vi "Add_spot_dialog_old.vi"(7 "Modify":bool, 8 "TransformedPt":bool, 9 "ArrayOfSpotNames":string[](array[string]), 10 "Current Session Information":T1={"CollectionOfPoints"=[{"MetaDataFile"=path "", "X"=0.0, "Y"=0.0, "Z"=0.0, "Group"=0, "Rotation"=0.0, "Fiducial"=FALSE, "Magnification"=0.0, "Working_Distance"=0.0, "Notes"="", "Location Name/ID"="", "OtherRelatedDataFiles"=[], "Available"=FALSE}, {"MetaDataFile"=path "", "X"=0.0, "Y"=0.0, "Z"=0.0, "Group"=0, "Rotation"=0.0, "Fiducial"=FALSE, "Magnification"=0.0, "Working_Distance"=0.0, "Notes"="", "Location Name/ID"="", "OtherRelatedDataFiles"=[], "Available"=FALSE}, {"MetaDataFile"=path "", "X"=0.0, "Y"=0.0, "Z"=0.0, "Group"=0, "Rotation"=0.0, "Fiducial"=FALSE, "Magnification"=0.0, "Working_Distance"=0.0, "Notes"="", "Location Name/ID"="", "OtherRelatedDataFiles"=[], "Available"=FALSE}, {"MetaDataFile"=path "", "X"=0.0, "Y"=0.0, "Z"=0.0, "Group"=0, "Rotation"=0.0, "Fiducial"=FALSE, "Magnification"=0.0, "Working_Distance"=0.0, "Notes"="", "Location Name/ID"="", "OtherRelatedDataFiles"=[], "Available"=FALSE}, {"MetaDataFile"=path "", "X"=0.0, "Y"=0.0, "Z"=0.0, "Group"=0, "Rotation"=0.0, "Fiducial"=FALSE, "Magnification"=0.0, "Working_Distance"=0.0, "Notes"="", "Location Name/ID"="", "OtherRelatedDataFiles"=[], "Available"=FALSE}, {"MetaDataFile"=path "", "X"=0.0, "Y"=0.0, "Z"=0.0, "Group"=0, "Rotation"=0.0, "Fiducial"=FALSE, "Magnification"=0.0, "Working_Distance"=0.0, "Notes"="", "Location Name/ID"="", "OtherRelatedDataFiles"=[], "Available"=FALSE}, {"MetaDataFile"=path "", "X"=0.0, "Y"=0.0, "Z"=0.0, "Group"=0, "Rotation"=0.0, "Fiducial"=FALSE, "Magnification"=0.0, "Working_Distance"=0.0, "Notes"="", "Location Name/ID"="", "OtherRelatedDataFiles"=[], "Available"=FALSE}], "Instrument"=enum."MXRD MFC", "CollectionFile"=path "/INL Macintosh/Users/timothymcjunkin/Desktop/Diffusion couple/MXRD 9-13-10/xrd_session_for_corrected.xml", "Session Name/ID"="xrd_test", "SessionNotes"="Sample moved to XRD"}, 11 "Input of Spot information":T2) -> (0 "Output of Spot information":T2, 1 "Current Session Information Out":T1={"CollectionOfPoints"=[{"MetaDataFile"=path "", "X"=0.0, "Y"=0.0, "Z"=0.0, "Group"=0, "Rotation"=0.0, "Fiducial"=FALSE, "Magnification"=0.0, "Working_Distance"=0.0, "Notes"="", "Location Name/ID"="", "OtherRelatedDataFiles"=[], "Available"=FALSE}, {"MetaDataFile"=path "", "X"=0.0, "Y"=0.0, "Z"=0.0, "Group"=0, "Rotation"=0.0, "Fiducial"=FALSE, "Magnification"=0.0, "Working_Distance"=0.0, "Notes"="", "Location Name/ID"="", "OtherRelatedDataFiles"=[], "Available"=FALSE}, {"MetaDataFile"=path "", "X"=0.0, "Y"=0.0, "Z"=0.0, "Group"=0, "Rotation"=0.0, "Fiducial"=FALSE, "Magnification"=0.0, "Working_Distance"=0.0, "Notes"="", "Location Name/ID"="", "OtherRelatedDataFiles"=[], "Available"=FALSE}, {"MetaDataFile"=path "", "X"=0.0, "Y"=0.0, "Z"=0.0, "Group"=0, "Rotation"=0.0, "Fiducial"=FALSE, "Magnification"=0.0, "Working_Distance"=0.0, "Notes"="", "Location Name/ID"="", "OtherRelatedDataFiles"=[], "Available"=FALSE}, {"MetaDataFile"=path "", "X"=0.0, "Y"=0.0, "Z"=0.0, "Group"=0, "Rotation"=0.0, "Fiducial"=FALSE, "Magnification"=0.0, "Working_Distance"=0.0, "Notes"="", "Location Name/ID"="", "OtherRelatedDataFiles"=[], "Available"=FALSE}, {"MetaDataFile"=path "", "X"=0.0, "Y"=0.0, "Z"=0.0, "Group"=0, "Rotation"=0.0, "Fiducial"=FALSE, "Magnification"=0.0, "Working_Distance"=0.0, "Notes"="", "Location Name/ID"="", "OtherRelatedDataFiles"=[], "Available"=FALSE}, {"MetaDataFile"=path "", "X"=0.0, "Y"=0.0, "Z"=0.0, "Group"=0, "Rotation"=0.0, "Fiducial"=FALSE, "Magnification"=0.0, "Working_Distance"=0.0, "Notes"="", "Location Name/ID"="", "OtherRelatedDataFiles"=[], "Available"=FALSE}], "Instrument"=enum."MXRD MFC", "CollectionFile"=path "/INL Macintosh/Users/timothymcjunkin/Desktop/Diffusion couple/MXRD 9-13-10/xrd_session_for_corrected.xml", "Session Name/ID"="xrd_test", "SessionNotes"="Sample moved to XRD"}, 3 "Cancel":bool)   [LabVIEW 2011]
doc: "Pressing any of the add modify spots buttons launches a multi-purpose dialog box which is reconfigured to parts of the dialog box the user interacts with in each mode. This effectively reuses a lot of code that would have needed to be duplicated for the different cases. In the process makes this one dialog box more complicated. This dialog also gets called after a spot from a previous session dialog box is completed. Two types of adds are possible without a calculation, one for a fiducial and one for a spot of interest that is not a fiducial. The modify version of this dialog box is simply supplied with the exiting information from a spot and allows the user to change the spot information. It may be called from the modify or the edit button on the sample information tab or the current session tab. The only difference is where the information comes from and goes to."
uses:
  cm2nm_coordinate_information_v2.ctl
  cm2nm_sample_set.ctl
  Instrument_type_enum_v2.ctl
  cm2nm_fiducial_selector.ctl
panel:
  in  "Allow_nonstandard_fids":bool
  out "error out 2":errorcluster
  in  "Cancel 2":bool
  out "Original_group":i32
  out "Instructions":string
  in  "Group Coding":i32
  out "MetaDataAvailable":bool caption="Is a Fiducial"
  out "error out":errorcluster
  in  "Notes:":string
  in  "Tab Control":T4(tab)
  in  "Fiducial Selector":T5
  in  "Tilt":dbl
  in  "Stage Rotation":dbl
  in  "Get Coordinates from Meta File":bool
  in  "Move to next screen":bool
  in  "Spot Name":string
  in  "Z-Position":dbl
  in  "Y-Position":dbl
  in  "X-Position":dbl
  in  "MetaDataFile":path
  in  "Cancel2":bool caption="Cancel"
  in  "Fiducial?":bool
  in  "Add A Spot Related Data File":bool caption="Add Another File\nRelated to this Spot"
  in  "Goto Previous Screen":bool caption="Press to Move to \nPrevious Screen"
  in  "Press to goto final Screen":bool caption="Press to Move to Next\nInformation Screen"
  out "OtherRelatedDataFiles":T6(array[cluster])
  in  "Cancel3":bool
  in  "Go Back to Correct":bool
  in  "AddToDataBase":bool
  # "Enter or confirm the\nspot  name and positions\n\nIf Metafile is available \nselect it in the MetaDatafile\nField and click Use MetaFile\nto extract MetaData\nFrom the file."
  # "This form allows you\nto add any number of\nfiles related to this\nspot on the sample.\nFor example spectra\nfiles or images other\nthan the file \ncontaining meta data."
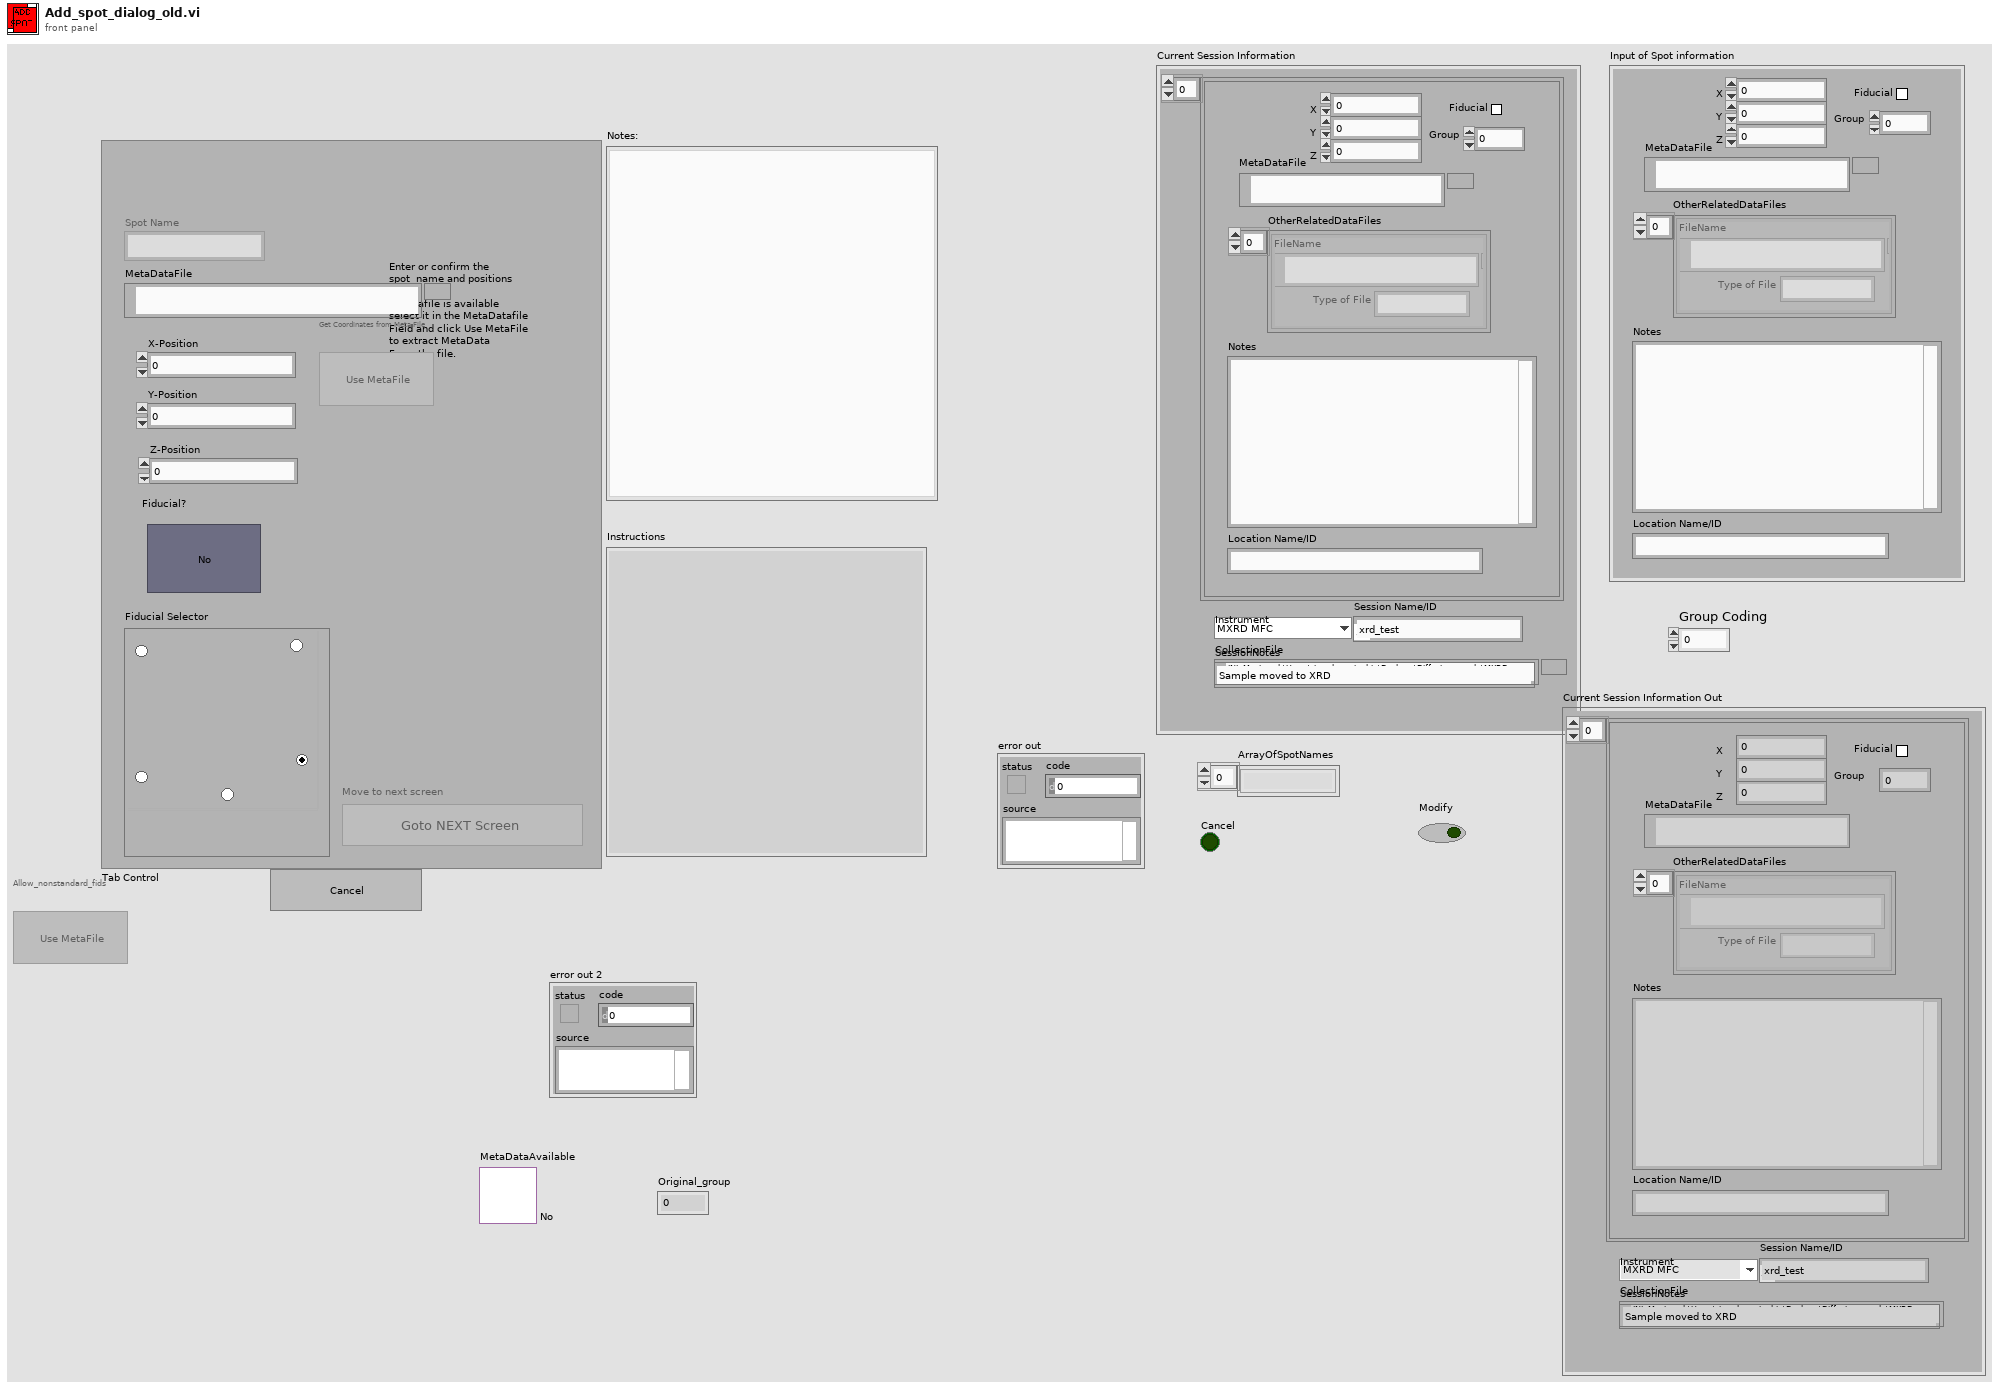
[diagram p1: front panel]
types:
  T1 = typedef "cm2nm_sample_set.ctl" = cluster{"CollectionOfPoints":T2[], "Instrument":T3, "CollectionFile":path, "Session Name/ID":string, "SessionNotes":string}
  T2 = typedef "cm2nm_coordinate_information_v2.ctl" = cluster{"MetaDataFile":path, "X":dbl, "Y":dbl, "Z":dbl, "Group":i32, "Rotation":dbl[unit], "Fiducial":bool, "Magnification":dbl, "Working_Distance":dbl, "Notes":string, "Location Name/ID":string, "OtherRelatedDataFiles":cluster{"Type of File":string, "FileName":path}[], "Available":bool}
  T3 = typedef "Instrument_type_enum_v2.ctl" = enum16{"Unknown", "Philips FEI SEM IRC", "JEOL 7000F EML_MFC", "MXRD MFC", "JEOL_EPMA"}
  T4 = enum32{"Name and Postions", "ExtraDataFiles", "SpotSummary"}
  T5 = typedef "cm2nm_fiducial_selector.ctl" = enum32{"Fiducial 1", "Fiducial 2", "Fiducial 3", "Fiducial 4", "Fiducial 5", "Other/NonStandard"}
  T6 = cluster{"Type of File":string, "FileName":path}[]
  T7 = enum8{"Enabled", "Disabled", "Disabled and Grayed Out"}
  T8 = enum32{"Name and Postions", "ExtraDataFiles", "SpotSummary", "Inputs"}
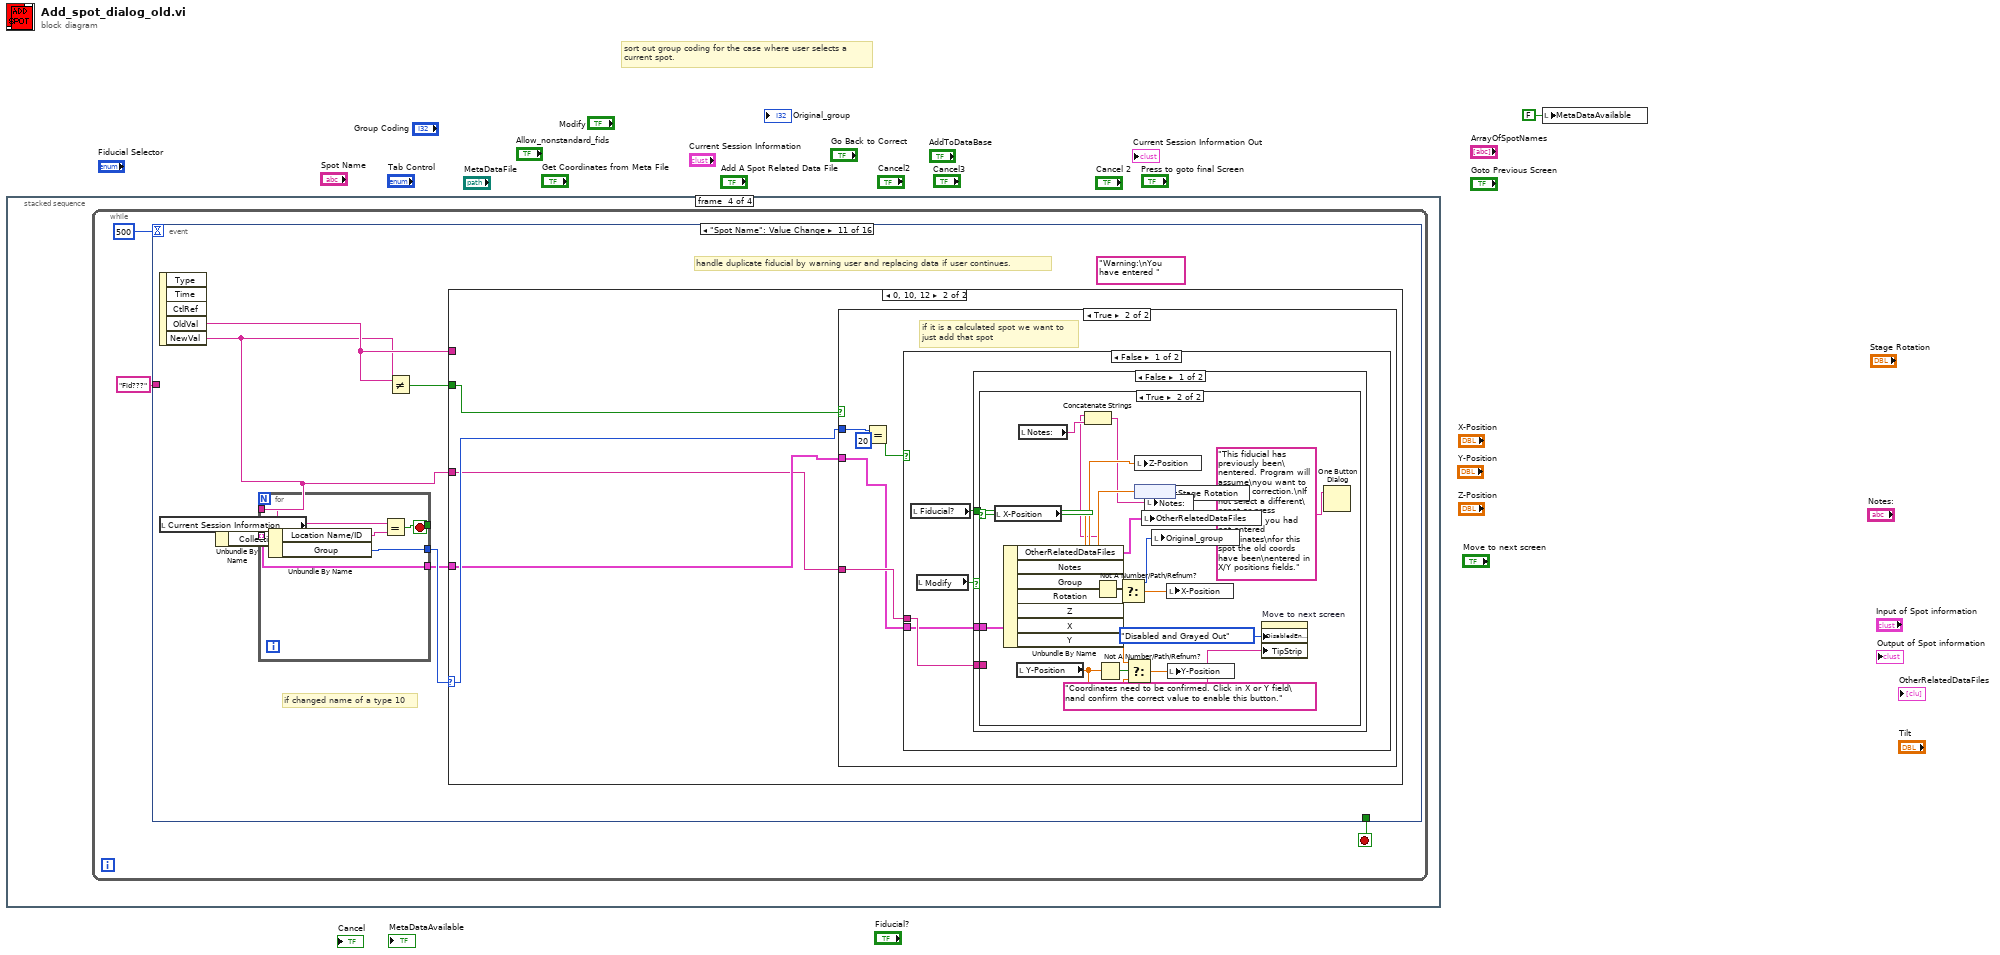
[diagram p0: block diagram]
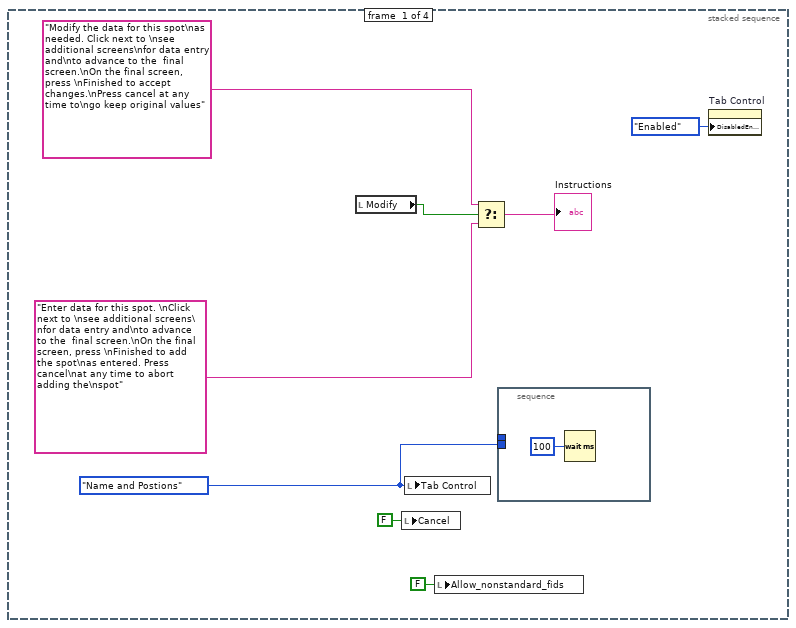
[diagram p2: hidden frame]
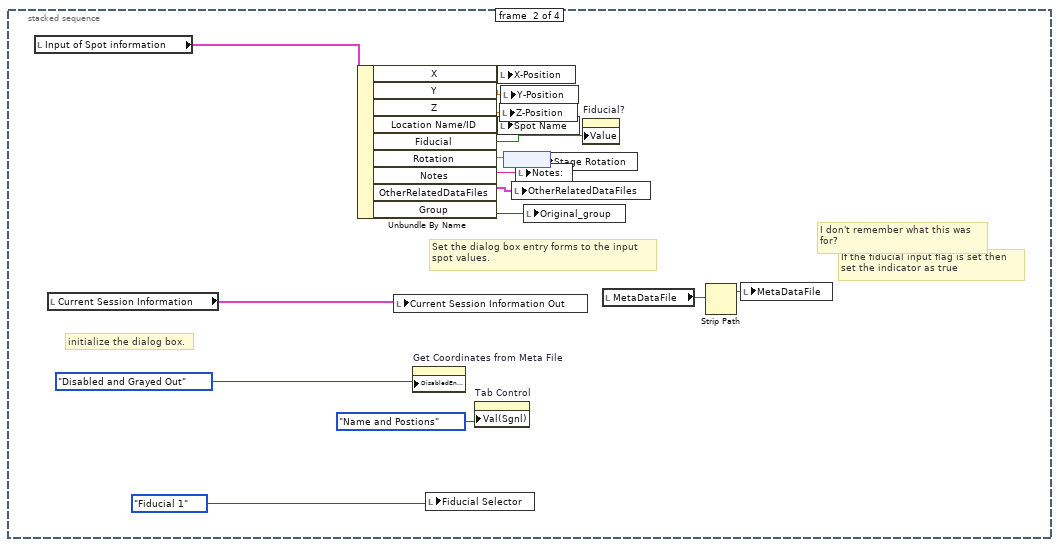
[diagram p3: hidden frame]
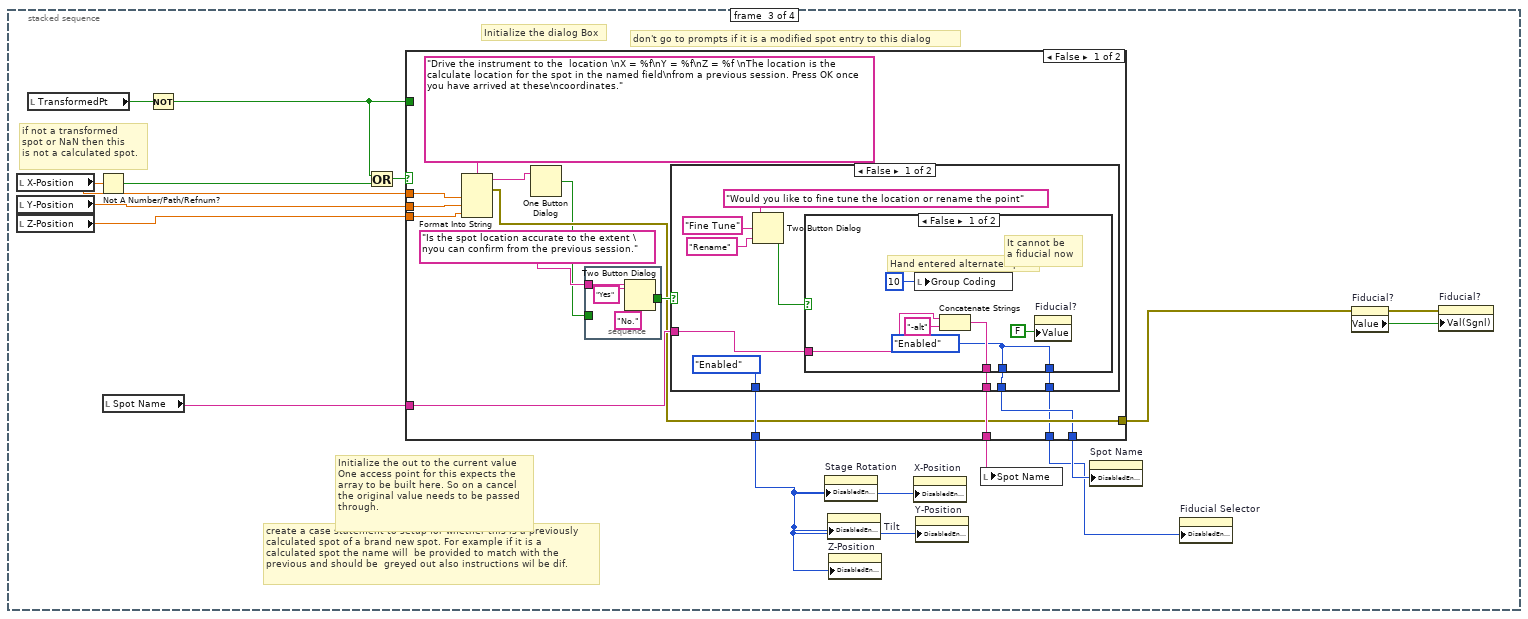
[diagram p4: hidden frame]
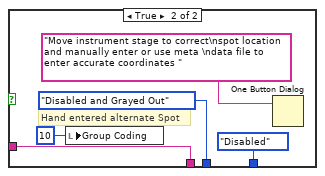
[diagram p5: hidden frame]
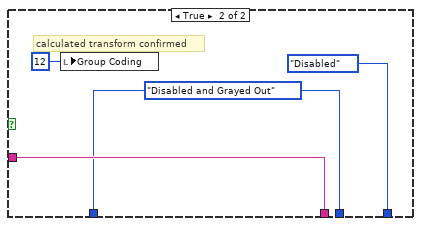
[diagram p6: hidden frame]
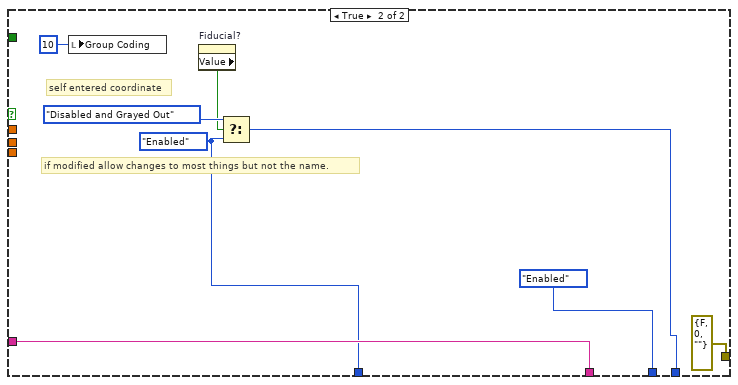
[diagram p7: hidden frame]
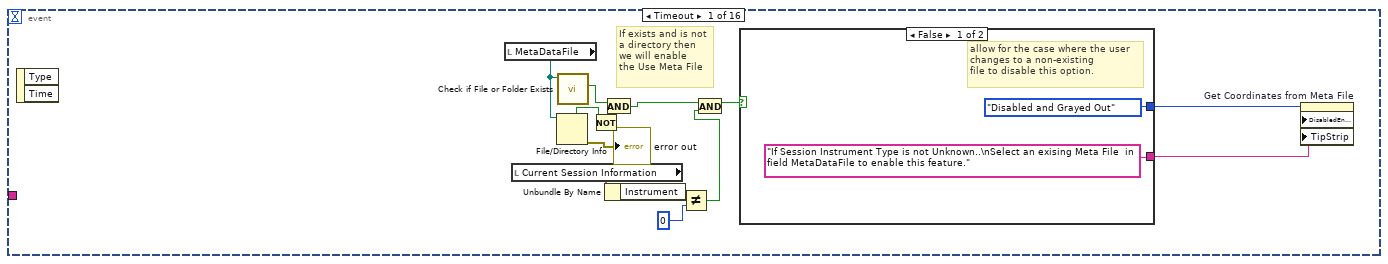
[diagram p8: hidden frame]
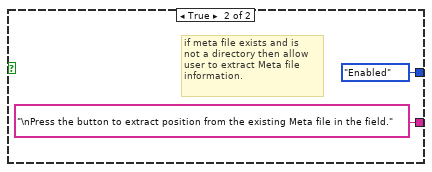
[diagram p9: hidden frame]
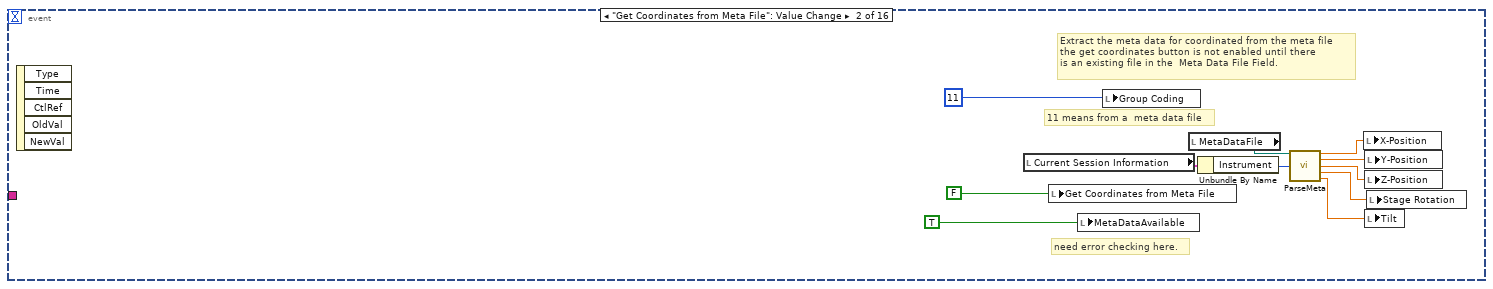
[diagram p10: hidden frame]
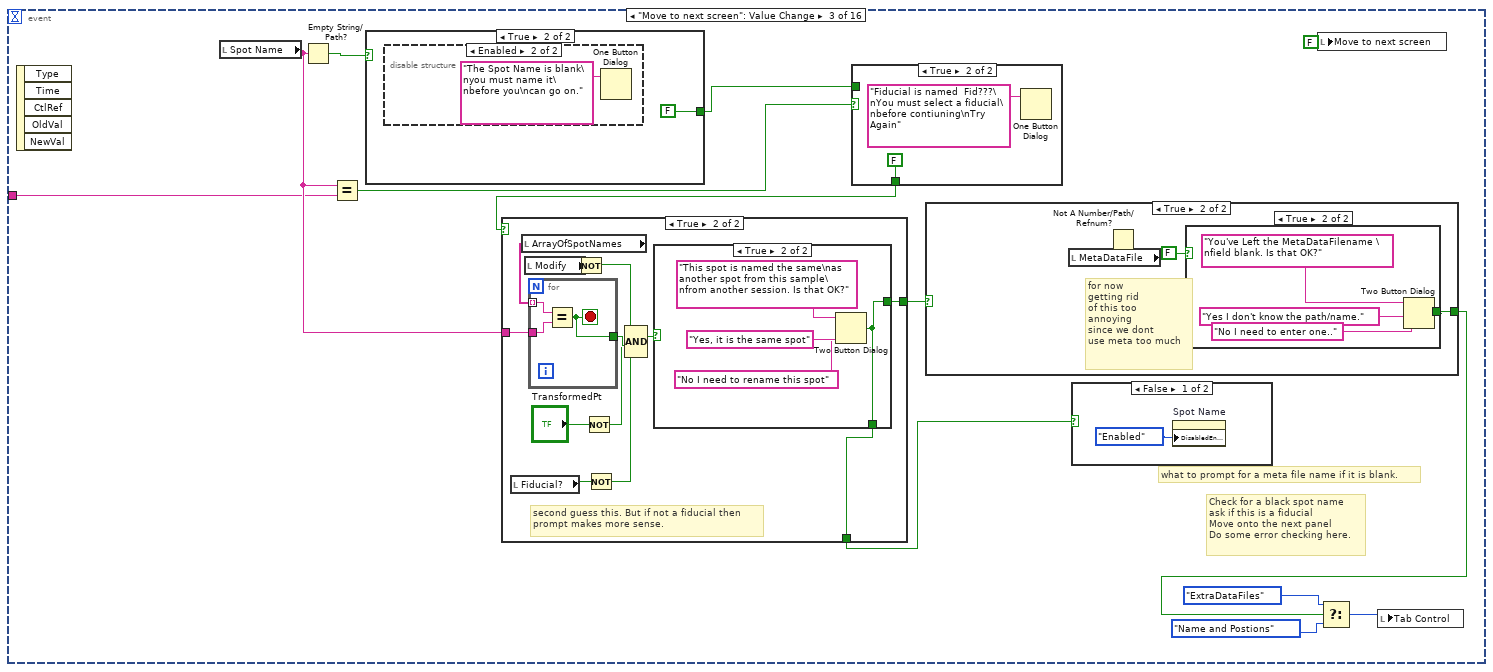
[diagram p11: hidden frame]
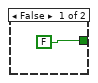
[diagram p14: hidden frame]
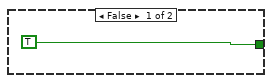
[diagram p15: hidden frame]
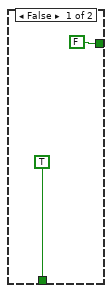
[diagram p16: hidden frame]
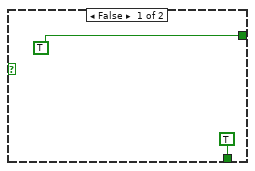
[diagram p17: hidden frame]
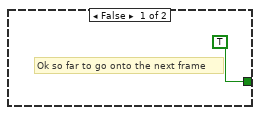
[diagram p18: hidden frame]
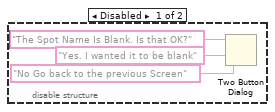
[diagram p19: hidden frame]
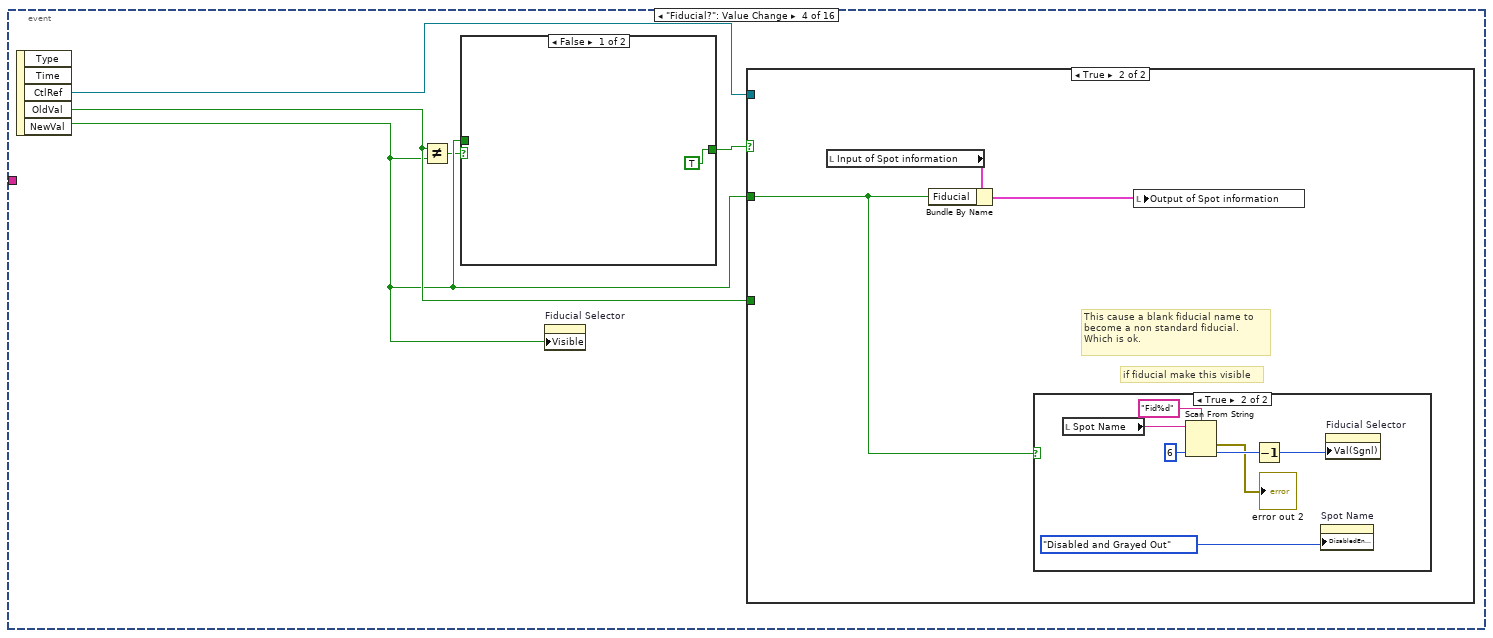
[diagram p20: hidden frame]
diagram:
  # "sort out group coding for the case where user selects a\ncurrent spot."
  n1 = stacked-sequence {
    frame #0 {
      w5 = T8."Name and Postions" ("Tab Control")
      n2 = local read "Modify"() -> (w6:bool)
      n3 = local write "Cancel"(FALSE ("Cancel")) -> ()
      n4 = local write "Tab Control"(w5) -> ()
      n5 = local write "Allow_nonstandard_fids"(FALSE ("Allow_nonstandard_fids")) -> ()
      n6 = Select(t="Modify the data for this spot\nas needed. Click next to \nsee additional screens\nfor data entry and\nto advance to the  final screen.\nOn the final screen, press \nFinished to accept changes.\nPress cancel at any time to\ngo keep original values" ("Instructions"), s=w6, f="Enter data for this spot. \nClick next to \nsee additional screens\nfor data entry and\nto advance to the  final screen.\nOn the final screen, press \nFinished to add the spot\nas entered. Press cancel\nat any time to abort adding the\nspot" ("Instructions")) -> (s? t:f=→"Instructions":string)
      n7 = stacked-sequence {
        tunnel: [w10] -> _
        tunnel: w5 -> [w10]
        frame #0 {
          n8 = Wait (ms)(milliseconds to wait=u32 100) -> ()  [unwired: 1 out]
        }
      }
      n9 = property on="Tab Control" class="TabCtl (strict)"("DisabledEnum"=T7."Enabled" ("Disabled")) -> ()  [unwired: 2 in, 2 out]
    }
    frame #1 {
      # "initialize the dialog box."
      # "I don't remember what this was\nfor?"
      # "If the fiducial input flag is set then \nset the indicator as true"
      # "Set the dialog box entry forms to the input\nspot values."
      n10 = local read "Input of Spot information"() -> (w28:T2)
      n11 = local read "Current Session Information"() -> (w19:T1)
      n12 = Unbundle By Name(w28) -> ("X"=w20:dbl, "Y"=w27:dbl, "Z"=w25:dbl, "Location Name/ID"=w26:string, "Fiducial"=w14:bool, "Rotation"=w24:dbl[unit], "Notes"=w22:string, "OtherRelatedDataFiles"=w21:T6, "Group"=w12:i32)
      n13 = local write "Current Session Information Out"(w19) -> ()
      n14 = property on="Get Coordinates from Meta File" class="Bool (strict)"("DisabledEnum"=T7."Disabled and Grayed Out" ("Disabled")) -> ()  [unwired: 2 in, 2 out]
      n15 = local write "Fiducial Selector"(cm2nm_fiducial_selector."Fiducial 1" ("Fiducial Selector")) -> ()
      n16 = property on="Tab Control" class="TabCtl (strict)"("Val(Sgnl)"=T8."Name and Postions" ("Tab Control")) -> ()  [unwired: 2 in, 2 out]
      n17 = local write "X-Position"(w20) -> ()
      n18 = local write "Spot Name"(w26) -> ()
      n19 = local write "Z-Position"(w25) -> ()
      n20 = local write "Y-Position"(w27) -> ()
      n21 = node(w24) -> (w23:dbl)
      n22 = local write "OtherRelatedDataFiles"(w21) -> ()
      n23 = local write "Notes:"(w22) -> ()
      n24 = local write "Original_group"(w12) -> ()
      n25 = local write "Stage Rotation"(w23) -> ()
      n26 = property on="Fiducial?" class="Bool (strict)"("Value"=w14) -> ()  [unwired: 2 in, 2 out]
      n27 = local read "MetaDataFile"() -> (w16:path)
      n28 = Strip Path(path=w16) -> (stripped path=w15:path)  [unwired: 1 out]
      n29 = local write "MetaDataFile"(w15) -> ()
    }
    frame #2 {
      # "if not a transformed\nspot or NaN then this\nis not a calculated spot."
      # "don't go to prompts if it is a modified spot entry to this dialog"
      # "Initialize the out to the current value\nOne access point for this expects the\narray to be built here. So on a cancel\nthe original value needs to be passed\nthrough."
      # "Initialize the dialog Box"
      # "create a case statement to setup for whether this is a previously\ncalculated spot of a brand new spot. For example if it is a\ncalculated spot the name will  be provided to match with the \nprevious and should be  greyed out also instructions wil be dif."
      n30 = local read "X-Position"() -> (w38:dbl)
      n31 = local read "Y-Position"() -> (w40:dbl)
      n32 = local read "Z-Position"() -> (w39:dbl)
      n33 = local read "TransformedPt"() -> (w31:bool)
      n34 = Not A Number/Path/Refnum?(number/path/refnum=w38) -> (NaN/Path/Refnum?=w36:bool)
      n35 = local read "Spot Name"() -> (w37:string)
      n36 = Not(x=w31) -> (.not. x?=w35:bool)
      n37 = Or(x=w35, y=w36) -> (x .or. y?=w41:bool)
      n38 = case shown="False" w41 {
        tunnel: [w50 w89] -> w43
        tunnel: w38 -> [w56 _]
        tunnel: w40 -> [w55 _]
        tunnel: [w45 w90] -> w30
        tunnel: w37 -> [w49 w93]
        tunnel: [w48 w93] -> w42
        tunnel: w39 -> [w52 _]
        tunnel: w35 -> [_ _]
        tunnel: [w47 errorcluster {"status"=FALSE, "code"=0, "source"=""} ("error IO")] -> w33
        tunnel: [w44 T7."Enabled" ("Disabled")] -> w29
        frame False {
          n39 = Format Into String(format string="Drive the instrument to the  location \nX = %f\nY = %f\nZ = %f \nThe location is the calculate location for the spot in the named field\nfrom a previous session. Press OK once you have arrived at these\ncoordinates.", w56, w55, w52) -> (resulting string=w54:string, error out=w47:errorcluster)  [unwired: 2 in]
          n40 = One Button Dialog ("Drive to the Calculated Coordinates")(message=w54) -> (true=w46:bool)  [unwired: 1 in]
          n41 = stacked-sequence {
            tunnel: "Is the spot location accurate to the extent \nyou can confirm from the previous session." -> [w61]
            tunnel: [w58] -> w51
            tunnel: w46 -> [_]
            frame #0 {
              n42 = Two Button Dialog(message=w61, 1:"No." ("F button name (\"Cancel\")"), 2:"Yes" ("T button name (\"OK\")")) -> (T button?=w58:bool)
            }
          }
          n43 = case shown="False" w51 {
            tunnel: [T7."Enabled" ("Disabled") w84] -> w50
            tunnel: w49 -> [w65 w85]
            tunnel: [w64 w85] -> w48
            tunnel: [w63 w84] -> w45
            tunnel: [w62 T7."Disabled" ("Disabled")] -> w44
            frame False {
              n44 = Two Button Dialog(message="Would you like to fine tune the location or rename the point", 1:"Rename" ("F button name (\"Cancel\")"), 2:"Fine Tune" ("T button name (\"OK\")")) -> (T button?=w66:bool)
              n45 = case shown="False" w66 {
                tunnel: w65 -> [w75 w81]
                tunnel: [w74 w81] -> w64
                tunnel: [w71 T7."Disabled and Grayed Out" ("Disabled")] -> w63
                tunnel: [w71 T7."Disabled" ("Disabled")] -> w62
                frame False {
                  w71 = T7."Enabled" ("Disabled")
                  # "It cannot be\na fiducial now"
                  # "Hand entered alternate Spot"
                  n46 = local write "Group Coding"(10 ("Group Coding")) -> ()
                  n47 = Concatenate Strings(w75, "-alt" ("string")) -> (w74:string)
                  n48 = property on="Fiducial?" class="Bool (strict)"("Value"=FALSE ("Fiducial?")) -> ()  [unwired: 2 in, 2 out]
                }
                frame True {
                  # "Hand entered alternate Spot"
                  n49 = local write "Group Coding"(10 ("Group Coding")) -> ()
                  n50 = One Button Dialog ("Drive to the Calculated Coordinates")(message="Move instrument stage to correct\nspot location and manually enter or use meta \ndata file to enter accurate coordinates ") -> ()  [unwired: 1 in, 1 out]
                }
              }
            }
            frame True {
              w84 = T7."Disabled and Grayed Out" ("Disabled")
              # "calculated transform confirmed"
              n51 = local write "Group Coding"(12 ("Group Coding")) -> ()
            }
          }
        }
        frame True {
          w89 = T7."Enabled" ("Disabled")
          # "if modified allow changes to most things but not the name."
          # "self entered coordinate"
          n52 = local write "Group Coding"(10 ("Group Coding")) -> ()
          n53 = property on="Fiducial?" class="Bool (strict)"() -> ("Value"=w87:bool)  [unwired: 2 in, 2 out]
          n54 = Select(t=T7."Disabled and Grayed Out" ("Disabled"), s=w87, f=w89) -> (s? t:f=w90:T7)
        }
      }
      n55 = property on="Stage Rotation" class="DigNum (strict)"("DisabledEnum"=w43) -> ()  [unwired: 2 in, 2 out]
      n56 = property on="Tilt" class="DigNum (strict)"("DisabledEnum"=w43) -> ()  [unwired: 2 in, 2 out]
      n57 = property on="Z-Position" class="DigNum (strict)"("DisabledEnum"=w43) -> ()  [unwired: 2 in, 2 out]
      n58 = property on="X-Position" class="DigNum (strict)"("DisabledEnum"=w43) -> ()  [unwired: 2 in, 2 out]
      n59 = property on="Y-Position" class="DigNum (strict)"("DisabledEnum"=w43) -> ()  [unwired: 2 in, 2 out]
      n60 = local write "Spot Name"(w42) -> ()
      n61 = property on="Spot Name" class="Str"("DisabledEnum"=w30) -> ()  [unwired: 2 in, 2 out]
      n62 = property on="Fiducial Selector" class="RadioBtnsControl (strict)"("DisabledEnum"=w29) -> ()  [unwired: 2 in, 2 out]
      n63 = property on="Fiducial?" class="Bool (strict)"(error in=w33) -> (error out=w34:errorcluster, "Value"=w32:bool)  [unwired: 1 in, 1 out]
      n64 = property on="Fiducial?" class="Bool (strict)"(error in=w34, "Val(Sgnl)"=w32) -> ()  [unwired: 1 in, 2 out]
    }
    frame #3 {
      n65 = while {
        stop <- w95 stop-if-true
        n66 = event shown="[10] \"Spot Name\": Value Change" {
          selector: _ -> [_ _ _ _ _ _ _ _ _ _ _ _ _ _ _ _]
          dyn-events: _ -> [_ _ _ _ _ _ _ _ _ _ _ _ _ _ _ _]
          timeout: 500 -> [_ _ _ _ _ _ _ _ _ _ _ _ _ _ _ _]
          tunnel: [_ _ _ _ _ TRUE ("T button?") w250 _ _ _ _ w362 _ _ _ _] -> w95
          tunnel: "Fid???" ("Value (Signaling)") -> [_ _ w128 _ w206 _ _ _ _ _ _ _ _ _ _ _]
          event Timeout {
            # "If exists and is not\na directory then\nwe will enable \nthe Use Meta File"
            n67 = event-data() -> ()  [unwired: 1 in, 2 out]
            n68 = local read "MetaDataFile"() -> (w102:path)
            n69 = local read "Current Session Information"() -> (w101:T1)
            n70 = File/Directory Info(path=w102) -> (directory=w109:bool, error out=→"error out":errorcluster)  [unwired: 1 in, 5 out]
            n71 = call <vilib>:"Check if File or Folder Exists.vi"("path"=w102) -> ("file or folder exists?"=w107:bool)  [unwired: 8 in, 2 out]
            n72 = Not(x=w109) -> (.not. x?=w108:bool)
            n73 = And(x=w107, y=w108) -> (x .and. y?=w103:bool)
            n74 = Unbundle By Name(w101) -> ("Instrument"=w100:T3)
            n75 = Not Equal?(x=w100, y=u16 0) -> (x != y?=w97:bool)
            n76 = And(x=w103, y=w97) -> (x .and. y?=w98:bool)
            n77 = case shown="False" w98 {
              tunnel: [T7."Disabled and Grayed Out" ("Disabled") T7."Enabled" ("Disabled")] -> w105
              tunnel: ["If Session Instrument Type is not Unknown..\nSelect an exising Meta File  in field MetaDataFile to enable this feature." ("Tip Strip") "\nPress the button to extract position from the existing Meta file in the field." ("Tip Strip")] -> w104
              frame False {
                # "allow for the case where the user\nchanges to a non-existing\nfile to disable this option."
              }
              frame True {
                # "if meta file exists and is\nnot a directory then allow \nuser to extract Meta file \ninformation."
              }
            }
            n78 = property on="Get Coordinates from Meta File" class="Bool (strict)"("DisabledEnum"=w105, "TipStrip"=w104) -> ()  [unwired: 2 in, 2 out]
          }
          event "Get Coordinates from Meta File": Value Change {
            # "11 means from a  meta data file"
            # "need error checking here."
            # "Extract the meta data for coordinated from the meta file\nthe get coordinates button is not enabled until there\nis an existing file in the  Meta Data File Field."
            n79 = event-data() -> ()  [unwired: 1 in, 5 out]
            n80 = local read "Current Session Information"() -> (w115:T1)
            n81 = local write "Get Coordinates from Meta File"(FALSE ("Get Coords")) -> ()
            n82 = local write "MetaDataAvailable"(TRUE ("MetaDataAvailable")) -> ()
            n83 = local write "Group Coding"(11 ("Group Coding")) -> ()
            n84 = local read "MetaDataFile"() -> (w123:path)
            n85 = Unbundle By Name(w115) -> ("Instrument"=w122:T3)
            n86 = call "ParseMeta.vi"("Path"=w123, "Instrument"=w122) -> ("X-stage (um)"=w121:dbl, "Y-stage (um)"=w120:dbl, "Z-stage (um)"=w119:dbl, "R-stage (deg)"=w118:dbl, "StageTilt"=w117:dbl)  [unwired: 1 in, 8 out]
            n87 = local write "X-Position"(w121) -> ()
            n88 = local write "Y-Position"(w120) -> ()
            n89 = local write "Z-Position"(w119) -> ()
            n90 = local write "Tilt"(w117) -> ()
            n91 = local write "Stage Rotation"(w118) -> ()
          }
          event "Move to next screen": Value Change {
            # "what to prompt for a meta file name if it is blank."
            # "Check for a black spot name\nask if this is a fiducial\nMove onto the next panel\nDo some error checking here."
            n92 = event-data() -> ()  [unwired: 1 in, 5 out]
            n93 = local read "Spot Name"() -> (w129:string)
            n94 = Empty String/Path?(string/path=w129) -> (empty?=w136:bool)
            n95 = Equal?(x=w129, y=w128) -> (x = y?=w127:bool)
            n96 = case shown="True" w136 {
              tunnel: [TRUE ("T button?") FALSE ("T button?")] -> w126
              frame False {
                # "Ok so far to go onto the next frame"
              }
              frame True {
                n97 = disable-structure shown="Enabled" {
                  frame Disabled {
                    n98 = Two Button Dialog(message="The Spot Name Is Blank. Is that OK?", 1:"No Go back to the previous Screen" ("F button name (\"Cancel\")"), 2:"Yes. I wanted it to be blank" ("T button name (\"OK\")")) -> ()  [unwired: 1 out]
                  }
                  frame Enabled {
                    n99 = One Button Dialog(message="The Spot Name is blank\nyou must name it\nbefore you\ncan go on.") -> ()  [unwired: 1 in, 1 out]
                  }
                }
              }
            }
            n100 = case shown="True" w127 {
              tunnel: w126 -> [w138 _]
              tunnel: [w138 FALSE ("T button?")] -> w125
              frame False {
              }
              frame True {
                n101 = One Button Dialog(message="Fiducial is named  Fid???\nYou must select a fiducial\nbefore contiuning\nTry Again") -> ()  [unwired: 1 in, 1 out]
              }
            }
            n102 = case shown="True" w125 {
              tunnel: w129 -> [_ w163]
              tunnel: [FALSE ("T button?") w161] -> w135
              tunnel: [TRUE ("T button?") w160] -> w130
              frame False {
              }
              frame True {
                # "second guess this. But if not a fiducial then \nprompt makes more sense."
                n103 = local read "Fiducial?"() -> (w154:bool)
                n104 = local read "ArrayOfSpotNames"() -> (w164:string[])
                n105 = local read "Modify"() -> (w155:bool)
                n106 = for {
                  tunnel: w164 -> [w173] mode=indexing
                  tunnel: w163 -> [w172]
                  tunnel: [w171] -> w162
                  stop <- w171 stop-if-true
                  n107 = Equal?(x=w173, y=w172) -> (x = y?=w171:bool)
                }
                n108 = Not(x=w155) -> (.not. x?=w156:bool)
                n109 = Not(x="TransformedPt") -> (.not. x?=w157:bool)
                n110 = Not(x=w154) -> (.not. x?=w153:bool)
                n111 = Compound Arithmetic op=AND(w156, w157, w162, w153) -> (w159:bool)
                n112 = case shown="True" w159 {
                  tunnel: [TRUE ("T button?") w167] -> w161
                  tunnel: [TRUE ("T button?") w167] -> w160
                  frame False {
                  }
                  frame True {
                    n113 = Two Button Dialog(message="This spot is named the same\nas another spot from this sample\nfrom another session. Is that OK?", 1:"No I need to rename this spot" ("F button name (\"Cancel\")"), 2:"Yes, it is the same spot" ("T button name (\"OK\")")) -> (T button?=w167:bool)
                  }
                }
              }
            }
            n114 = case shown="True" w135 {
              tunnel: [FALSE ("T button?") w144] -> w131
              frame False {
              }
              frame True {
                # "for now\ngetting rid \nof this too\nannoying\nsince we dont\nuse meta too much"
                n115 = local read "MetaDataFile"() -> (w145:path)
                n116 = Not A Number/Path/Refnum?(number/path/refnum=w145) -> ()  [unwired: 1 out]
                n117 = case shown="True" FALSE {
                  tunnel: [TRUE ("T button?") w147] -> w144
                  frame False {
                  }
                  frame True {
                    n118 = Two Button Dialog(message="You've Left the MetaDataFilename \nfield blank. Is that OK?", 1:"No I need to enter one.." ("F button name (\"Cancel\")"), 2:"Yes I don't know the path/name." ("T button name (\"OK\")")) -> (T button?=w147:bool)
                  }
                }
              }
            }
            n119 = case shown="False" w130 {
              frame False {
                n120 = property on="Spot Name" class="Str"("DisabledEnum"=T7."Enabled" ("Disabled")) -> ()  [unwired: 2 in, 2 out]
              }
              frame True {
              }
            }
            n121 = local write "Move to next screen"(FALSE ("Press to Move to Next\nInformation Screen")) -> ()
            n122 = Select(t=T8."ExtraDataFiles" ("Tab Control"), s=w131, f=T8."Name and Postions" ("Tab Control")) -> (s? t:f=w134:T8)
            n123 = local write "Tab Control"(w134) -> ()
          }
          event "Fiducial?": Value Change {
            n124 = event-data() -> ("CtlRef"=w180:refnum<vi>, "OldVal"=w183:bool, "NewVal"=w182:bool)  [unwired: 1 in, 2 out]
            n125 = Not Equal?(x=w183, y=w182) -> (x != y?=w181:bool)
            n126 = case shown="False" w181 {
              tunnel: [TRUE ("T button?") w187] -> w184
              tunnel: w182 -> [_ w186]
              frame False {
              }
              frame True {
                n127 = Select(t="You have changed this\nspot to be a fiducial.\nIs this correct?" ("message"), s=w186, f="You have changed this\nspot to NOT be a fiducial.\nIs this correct?\nIf YES please check the verify the Spot Name." ("message")) -> (s? t:f=w190:string)
                n128 = Two Button Dialog(message=w190, 1:"No" ("F button name (\"Cancel\")"), 2:"Yes" ("T button name (\"OK\")")) -> (T button?=w187:bool)
              }
            }
            n129 = property on="Fiducial Selector" class="RadioBtnsControl (strict)"("Visible"=w182) -> ()  [unwired: 2 in, 2 out]
            n130 = case shown="True" w184 {
              tunnel: w180 -> [w195 _]
              tunnel: w183 -> [w194 _]
              tunnel: w182 -> [_ w196]
              frame False {
                n131 = property class="Bool (strict)"(reference=w195, "Value"=w194) -> ()  [unwired: 1 in, 2 out]
                n132 = property on="Spot Name" class="Str"("DisabledEnum"=T7."Enabled" ("Disabled")) -> ()  [unwired: 2 in, 2 out]
              }
              frame True {
                # "This cause a blank fiducial name to\nbecome a non standard fiducial.\nWhich is ok."
                # "if fiducial make this visible"
                n133 = local read "Input of Spot information"() -> (w197:T2)
                n134 = Bundle By Name(cluster=w197, "Fiducial"=w196) -> (w198:T2)
                n135 = case shown="True" w196 {
                  frame False {
                  }
                  frame True {
                    n136 = local read "Spot Name"() -> (w205:string)
                    n137 = Scan From String(format string="Fid%d", input string=w205, default 1=6 ("default value 1")) -> (error out=→"error out 2":errorcluster, output 1=w202:i32)  [unwired: 2 in, 2 out]
                    n138 = Decrement(x=w202) -> (x-1=w201:i32)
                    n139 = property on="Spot Name" class="Str"("DisabledEnum"=T7."Disabled and Grayed Out" ("Disabled")) -> ()  [unwired: 2 in, 2 out]
                    n140 = property on="Fiducial Selector" class="RadioBtnsControl (strict)"("Val(Sgnl)"=w201) -> ()  [unwired: 2 in, 2 out]
                  }
                }
                n141 = local write "Output of Spot information"(w198) -> ()
              }
            }
          }
          event Value Change {
            n142 = event-data() -> ("NewVal"=w208:T5)  [unwired: 1 in, 4 out]
            n143 = Greater?(x=w208, y=cm2nm_fiducial_selector."Fiducial 5" ("Fiducial Selector")) -> (0:w210:bool)
            n144 = case shown="False" w210 {
              tunnel: w208 -> [w215 _]
              tunnel: [T7."Disabled and Grayed Out" ("Disabled") T7."Enabled" ("Disabled")] -> w207
              tunnel: w206 -> [_ w216]
              frame False {
                # "signal value change to check\nthe fiducial for duplicates."
                # "Auto assign the fiducial name."
                n145 = Increment(x=w215) -> (x+1=w214:T5)
                n146 = Format Into String(format string="Fid%d", w214) -> (resulting string=w211:string)  [unwired: 2 in, 1 out]
                n147 = property on="Spot Name" class="Str"("Val(Sgnl)"=w211) -> ()  [unwired: 2 in, 2 out]
              }
              frame True {
                n148 = property on="Spot Name" class="Str"("Val(Sgnl)"=w216) -> ()  [unwired: 2 in, 2 out]
                n149 = disable-structure shown="Disabled" {
                  frame Disabled {
                    n150 = One Button Dialog(message="Current Spot Name is a for\na non-standard\nFiducial\nDouble check\nthe Spot Name") -> ()  [unwired: 1 in, 1 out]
                  }
                  frame Enabled {
                  }
                }
              }
            }
            n151 = property on="Spot Name" class="Str"("DisabledEnum"=w207) -> ()  [unwired: 2 in, 2 out]
          }
          event "AddToDataBase": Value Change {
            # "Add it to this array"
            n152 = event-data() -> ()  [unwired: 1 in, 5 out]
            n153 = local read "Current Session Information"() -> (w220:T1)
            n154 = local read "Output of Spot information"() -> (w223:T2)
            n155 = Unbundle By Name(w220) -> ("CollectionOfPoints"=w224:T2[])
            n156 = local read "Modify"() -> (w221:bool)
            n157 = case shown="True" w221 {
              tunnel: w224 -> [w230 w234]
              tunnel: w223 -> [w229 w232]
              tunnel: [w228 w231] -> w222
              frame False {
                n158 = Build Array (concatenate)(w230, w229) -> (w228:T2[])
              }
              frame True {
                n159 = Unbundle By Name(w232) -> ("Location Name/ID"=w236:string)
                n160 = for {
                  tunnel: w234 -> [w248] mode=indexing
                  tunnel: w236 -> [w246]
                  tunnel: [w245] -> w235
                  tunnel: [w244] -> w233
                  i -> [w244]
                  stop <- w245 stop-if-true
                  n161 = Unbundle By Name(w248) -> ("Location Name/ID"=w247:string)
                  n162 = Equal?(x=w247, y=w246) -> (x = y?=w245:bool)
                }
                n163 = case shown="False" w235 {
                  tunnel: w234 -> [w239 w243]
                  tunnel: w233 -> [_ w242]
                  tunnel: w232 -> [w238 w241]
                  tunnel: [w237 w240] -> w231
                  frame False {
                    # "This means the name \nwas changed so add it"
                    n164 = Build Array (concatenate)(w239, w238) -> (w237:T2[])
                  }
                  frame True {
                    n165 = Replace Array Subset(array=w243, new element=w241, index=w242) -> (w240:T2[])
                  }
                }
              }
            }
            n166 = Bundle By Name(cluster=w220, "CollectionOfPoints"=w222) -> (w219:T1)
            n167 = stacked-sequence {
              tunnel: w219 -> [_]
              frame #0 {
                n168 = local write "Tab Control"(T4."Name and Postions" ("Tab Control")) -> ()
              }
            }
            n169 = local write "Current Session Information Out"(w219) -> ()
            n170 = local write "AddToDataBase"(FALSE ("AddToDataBase")) -> ()
          }
          event Panel Close? {
            w251 = FALSE ("Cancel")
            # "Give user one more chance to not cancel."
            n171 = event-data() -> ()  [unwired: 1 in, 3 out]
            n172 = Two Button Dialog(message="You have selected cancel adding this spot to the DataBase. Press \"Yes\" if that's what you intended.", 1:"Don't Cancel this Spot" ("F button name (\"Cancel\")"), 2:"YES. do not save this spot" ("T button name (\"OK\")")) -> (T button?=w250:bool)
            n173 = local write "Cancel"(w250) -> ()
            n174 = local write "Cancel 2"(w251) -> ()
            n175 = local write "Cancel2"(w251) -> ()
            n176 = local write "Cancel3"(w251) -> ()
            n177 = event-data("Discard?"=TRUE) -> ()  [unwired: 1 in, 1 out]
          }
          event "Goto Previous Screen": Value Change {
            n178 = event-data() -> ()  [unwired: 1 in, 5 out]
            n179 = local write "Goto Previous Screen"(FALSE ("Goto Previous Screen")) -> ()
            n180 = local write "Tab Control"(T8."Name and Postions" ("Tab Control")) -> ()
          }
          event "X-Position", "Y-Position", "Z-Position", "MetaDataFile": Value Change {
            # "If user changes any of these from the interface then the values did not come\nfrom the meta file and the indicator should be false."
            n181 = event-data() -> ("CtlRef"=w257:refnum<vi>, "OldVal"=w259:variant, "NewVal"=w258:variant)  [unwired: 1 in, 2 out]
            n182 = local read "Group Coding"() -> (w260:i32)
            n183 = case shown="11, 20" w260 {
              tunnel: w259 -> [_ _ w261]
              tunnel: w258 -> [_ _ _]
              tunnel: w257 -> [_ _ w262]
              frame 0, Default {
              }
              frame 10 {
                # "10 is ok  self entered no warning message for entering these values."
              }
              frame 11, 20 {
                # "coding from meta data file"
                n184 = Two Button Dialog(message="You have modified values\nread from the meta data\nfile or the meta data file name\n. Do you want to do \nthis?  ", 1:"No revert to the old meta data Value" ("F button name (\"Cancel\")"), 2:"Yes, keep the new values" ("T button name (\"OK\")")) -> (T button?=w263:bool)
                n185 = case shown="True" w263 {
                  tunnel: w262 -> [w267 _]
                  tunnel: w261 -> [w268 _]
                  frame False {
                    n186 = property class="Ctl"(reference=w267, "Value"=w268) -> ()  [unwired: 1 in, 2 out]
                  }
                  frame True {
                    # "change to 10 so the user\ncan modify as needed"
                    n187 = local write "Group Coding"(10 ("Group Coding")) -> ()
                  }
                }
              }
            }
          }
          event "X-Position", "Y-Position", "Z-Position": Mouse Enter {
            # "check for not a number. We do this here because the button may have been disabled\ndue to reselection of a repeated fiducial. User is required to touch one of the x/y/z\nfield to continue."
            n188 = event-data() -> ()  [unwired: 1 in, 3 out]
            n189 = local read "X-Position"() -> (w274:dbl)
            n190 = local read "Y-Position"() -> (w273:dbl)
            n191 = Not A Number/Path/Refnum?(number/path/refnum=w273) -> (NaN/Path/Refnum?=w271:bool)
            n192 = Not A Number/Path/Refnum?(number/path/refnum=w274) -> (NaN/Path/Refnum?=w272:bool)
            n193 = Or(x=w272, y=w271) -> (x .or. y?=w270:bool)
            n194 = case shown="False" w270 {
              tunnel: [T7."Enabled" ("Disabled") T7."Disabled and Grayed Out" ("Disabled")] -> w276
              tunnel: ["Click Next Once All Fields on this page are entered correctly" ("Tip Strip") "Enter valid numbers in X and Y Position to Continue" ("Tip Strip")] -> w275
              frame False {
              }
              frame True {
                # "allow for the case where the user\nchanges to a non-existing\nfile to disable this option."
              }
            }
            n195 = property on="Move to next screen" class="Bool (strict)"("DisabledEnum"=w276, "TipStrip"=w275) -> ()  [unwired: 2 in, 2 out]
          }
          event "Spot Name": Value Change {
            (unwired) "Warning:\nYou have entered "
            # "if changed name of a type 10"
            # "handle duplicate fiducial by warning user and replacing data if user continues."
            n196 = event-data() -> ("OldVal"=w287:string, "NewVal"=w281:string)  [unwired: 1 in, 3 out]
            n197 = local read "Current Session Information"() -> (w285:T1)
            n198 = Unbundle By Name(w285) -> ("CollectionOfPoints"=w284:T2[])
            n199 = for {
              tunnel: w284 -> [w288] mode=indexing
              tunnel: w281 -> [w291]
              tunnel: [w290] -> _
              tunnel: [w289] -> w283
              tunnel: [w288] -> w282
              stop <- w290 stop-if-true
              n200 = Unbundle By Name(w288) -> ("Location Name/ID"=w292:string, "Group"=w289:i32)
              n201 = Equal?(x=w291, y=w292) -> (x = y?=w290:bool)
            }
            n202 = Not Equal?(x=w287, y=w281) -> (x != y?=w286:bool)
            n203 = case shown="0, 10, 12" w283 {
              selector: w283 -> [_ w306]
              tunnel: w287 -> [w294 _]
              tunnel: w286 -> [w293 w304]
              tunnel: w282 -> [_ w305]
              tunnel: w281 -> [_ w303]
              frame 20, Default {
                # "need to check for a duplicate and\nreplace with the value."
                n204 = case shown="True" w293 {
                  tunnel: w294 -> [_ w295]
                  frame False {
                  }
                  frame True {
                    n205 = Two Button Dialog(message="You have changed a spot name of a point.\nassociated with other points in\nthe data base.\nDid you mean to do this?", 1:"No. Revert to the old name." ("F button name (\"Cancel\")"), 2:"Yes." ("T button name (\"OK\")")) -> (T button?=w296:bool)
                    n206 = case shown="True" w296 {
                      tunnel: w295 -> [w300 _]
                      frame False {
                        n207 = property on="Spot Name" class="Str"("Value"=w300) -> ()  [unwired: 2 in, 2 out]
                      }
                      frame True {
                        w301 = 10 ("Original_group")
                        n208 = local write "Group Coding"(w301) -> ()
                        n209 = local write "Original_group"(w301) -> ()
                        n210 = One Button Dialog(message="The old point will be\nkept in the database\nof this session. You may\nstill press cancel to leave\nthe database as it was.") -> ()  [unwired: 1 in, 1 out]
                      }
                    }
                  }
                }
              }
              frame 0, 10, 12 {
                n211 = case shown="True" w304 {
                  tunnel: w303 -> [_ w311]
                  tunnel: w306 -> [_ w310]
                  tunnel: w305 -> [_ w307]
                  frame False {
                  }
                  frame True {
                    # "if it is a calculated spot we want to\njust add that spot"
                    n212 = Equal?(x=w310, y=20) -> (x = y?=w308:bool)
                    n213 = case shown="False" w308 {
                      tunnel: w311 -> [w315 _]
                      tunnel: w307 -> [w312 w360]
                      frame False {
                        n214 = local read "Fiducial?"() -> (w313:bool)
                        n215 = local read "Modify"() -> (w314:bool)
                        n216 = case shown="False" w314 {
                          tunnel: w315 -> [w318 _]
                          tunnel: w313 -> [w317 _]
                          tunnel: w312 -> [w316 _]
                          frame False {
                            n217 = case shown="True" w317 {
                              tunnel: w318 -> [w321 _]
                              tunnel: w316 -> [_ w348]
                              frame False {
                                n218 = Random Number (0-1)() -> (number: 0 to 1=w329:dbl)
                                n219 = Multiply(x=w329, y=10000) -> (x*y=w325:dbl)
                                n220 = Round Toward -Infinity(1:w325) -> (0:w324:dbl)
                                n221 = To Unsigned Long Integer(number=w324) -> (unsigned 32bit integer=w323:u32)
                                n222 = Format Into String(w323) -> (resulting string=w326:string)  [unwired: 3 in, 1 out]
                                n223 = One Button Dialog(message="You have chosen a spot name that duplicates one in this session. \nA random number has been appended to it. to make it unique. \nIf you intended to modify an existing spot, cancel this dialog and select the spot in the current session tab drop down and press modify.") -> ()  [unwired: 1 in, 1 out]
                                n224 = Concatenate Strings(w321, "-" ("string"), w326) -> (w327:string)
                                n225 = property on="Spot Name" class="Str"("Val(Sgnl)"=w327, "DisabledEnum"=T7."Enabled" ("Disabled")) -> ()  [unwired: 2 in, 2 out]
                              }
                              frame True {
                                n226 = local read "X-Position"() -> (w341:dbl)
                                n227 = Unbundle By Name(w348) -> ("OtherRelatedDataFiles"=w331:T6, "Notes"=w333:string, "Group"=w330:i32, "Rotation"=w335:dbl[unit], "Z"=w336:dbl, "X"=w342:dbl, "Y"=w345:dbl)
                                n228 = local read "Y-Position"() -> (w343:dbl)
                                n229 = local read "Notes:"() -> (w334:string)
                                n230 = Concatenate Strings(w333, w334) -> (w332:string)
                                n231 = Not A Number/Path/Refnum?(number/path/refnum=w341) -> (NaN/Path/Refnum?=w347:bool)
                                n232 = Not A Number/Path/Refnum?(number/path/refnum=w343) -> (NaN/Path/Refnum?=w346:bool)
                                n233 = Select(t=w342, s=w347, f=w341) -> (s? t:f=w340:dbl)
                                n234 = Select(t=w345, s=w346, f=w343) -> (s? t:f=w344:dbl)
                                n235 = local write "Z-Position"(w336) -> ()
                                n236 = node(w335) -> (w337:dbl)
                                n237 = local write "OtherRelatedDataFiles"(w331) -> ()
                                n238 = local write "Notes:"(w332) -> ()
                                n239 = local write "Original_group"(w330) -> ()
                                n240 = local write "Stage Rotation"(w337) -> ()
                                n241 = local write "X-Position"(w340) -> ()
                                n242 = local write "Y-Position"(w344) -> ()
                                n243 = property on="Move to next screen" class="Bool (strict)"("DisabledEnum"=T7."Disabled and Grayed Out" ("Disabled"), "TipStrip"="Coordinates need to be confirmed. Click in X or Y field\nand confirm the correct value to enable this button." ("Tip Strip")) -> ()  [unwired: 2 in, 2 out]
                                n244 = One Button Dialog(message="This fiducial has previously been\nentered. Program will assume\nyou want to make a correction.\nIf not select a different\nspot or press cancel. \nIf you had not entered coordinates\nfor this spot the old coords have been\nentered in X/Y positions fields.") -> ()  [unwired: 1 in, 1 out]
                              }
                            }
                          }
                          frame True {
                            # "Dont error on modify on spot name if\nthe  name is the same. It should be."
                          }
                        }
                      }
                      frame True {
                        # "Was Calculated."
                        # "calculated transform confirmed"
                        # "convert this to a modify"
                        n245 = Unbundle By Name(w360) -> ("X"=w352:dbl, "Y"=w351:dbl, "Z"=w350:dbl, "Notes"=w358:string)
                        n246 = local write "Modify"(TRUE ("Modify")) -> ()
                        n247 = local read "Notes:"() -> (w359:string)
                        n248 = Concatenate Strings(w358, w359) -> (w357:string)
                        n249 = local write "X-Position"(w352) -> ()
                        n250 = local write "Z-Position"(w350) -> ()
                        n251 = local write "Y-Position"(w351) -> ()
                        n252 = property on="Notes:" class="Str"("Val(Sgnl)"=w357) -> ()  [unwired: 2 in, 2 out]
                        n253 = local write "Group Coding"(12 ("Group Coding")) -> ()
                        n254 = Format Into String(format string="Enough fiducials have been entered to calculate the position\nof this spot. The calcuated position for this spot is:\nX = %f\nY = %f\nZ = %f \nThe value of the coordinates has been transfered to the\nAdd Spot Dialog box for you convenience.  You may correct\nthe position.", w352, w351, w350) -> (resulting string=w353:string)  [unwired: 2 in, 1 out]
                        n255 = One Button Dialog ("Drive to the Calculated Coordinates")(message=w353) -> ()  [unwired: 1 in, 1 out]
                      }
                    }
                  }
                }
              }
            }
          }
          event "Cancel2", "Cancel3", "Cancel 2": Value Change {
            w361 = FALSE ("Cancel")
            n256 = event-data() -> ()  [unwired: 1 in, 5 out]
            n257 = local write "Cancel 2"(w361) -> ()
            n258 = local write "Cancel2"(w361) -> ()
            n259 = local write "Cancel3"(w361) -> ()
            n260 = Two Button Dialog(message="You have selected cancel adding this spot to the DataBase. Press \"Yes\" if that's what you intended.", 1:"Don't Cancel this Spot" ("F button name (\"Cancel\")"), 2:"YES. do not save this spot" ("T button name (\"OK\")")) -> (T button?=w362:bool)
            n261 = local write "Cancel"(w362) -> ()
          }
          event "Add A Spot Related Data File": Value Change {
            # "prompt user for adding\na file"
            n262 = event-data() -> ()  [unwired: 1 in, 5 out]
            n263 = local read "OtherRelatedDataFiles"() -> (w368:T6)
            n264 = Array Size(array=w368) -> (size(s)=w367:i32)
            n265 = Greater Than 0?(x=w367) -> (x > 0?=w369:bool)
            n266 = case shown="False" w369 {
              tunnel: w368 -> [_ w377]
              tunnel: w367 -> [_ w379]
              tunnel: [path "" w375] -> w366
              frame False {
              }
              frame True {
                n267 = Decrement(x=w379) -> (x-1=w378:i32)
                n268 = Index Array(array=w377, index=w378) -> (element=w376:cluster{"Type of File":string, "FileName":path})
                n269 = Unbundle By Name(w376) -> ("FileName"=w375:path)
              }
            }
            n270 = call "Add_related_file.vi"("Path"=w366) -> ("Type or Description of File Out"=w371:string, "Path_out"=w372:path, "Cancelled?"=w373:bool)  [unwired: 8 in]
            n271 = case shown="False" w373 {
              tunnel: w372 -> [w384 _]
              tunnel: w371 -> [w383 _]
              tunnel: w368 -> [w380 _]
              frame False {
                n272 = Bundle By Name(cluster=cluster{"Type of File":string, "FileName":path} {"Type of File"="", "FileName"=path ""} ("element"), "FileName"=w384, "Type of File"=w383) -> (w382:cluster{"Type of File":string, "FileName":path})
                n273 = Build Array (concatenate)(w380, w382) -> (w381:T6)
                n274 = local write "OtherRelatedDataFiles"(w381) -> ()
              }
              frame True {
              }
            }
            n275 = local write "Add A Spot Related Data File"(FALSE ("Add A Spot Related Data File")) -> ()
          }
          event "Press to goto final Screen", "Tab Control": Value Change {
            w392 = 0.0 ("Magnification")
            # "new coding on group\n10 - is a user entered item"
            n276 = event-data() -> ("CtlRef"=w389:refnum<vi>)  [unwired: 1 in, 4 out]
            n277 = local read "OtherRelatedDataFiles"() -> (w393:T6)
            n278 = local read "Stage Rotation"() -> (w399:dbl)
            n279 = local read "X-Position"() -> (w401:dbl)
            n280 = local read "Y-Position"() -> (w402:dbl)
            n281 = local read "Z-Position"() -> (w400:dbl)
            n282 = local read "MetaDataAvailable"() -> (w396:bool)
            n283 = local read "Group Coding"() -> (w391:i32)
            n284 = local read "MetaDataFile"() -> (w403:path)
            n285 = local read "Spot Name"() -> (w394:string)
            n286 = property class="Ctl"(reference=w389) -> ("Label.Text"=w388:string)  [unwired: 1 in, 2 out]
            n287 = local read "Fiducial?"() -> (w397:bool)
            n288 = local read "Notes:"() -> (w395:string)
            n289 = node(w399) -> (w398:dbl[unit])
            n290 = local read "Input of Spot information"() -> (w390:T2)
            n291 = Equal?(x=w388, y="Press to goto final Screen") -> (x = y?=w386:bool)
            n292 = Bundle By Name(cluster=w390, "MetaDataFile"=w403, "X"=w401, "Y"=w402, "Group"=w391, "Z"=w400, "Rotation"=w398, "Fiducial"=w397, "Magnification"=w392, "Working_Distance"=w392, "Notes"=w395, "Location Name/ID"=w394, "OtherRelatedDataFiles"=w393, "Available"=w396) -> (w404:T2)
            n293 = case shown="True" w386 {
              frame False {
              }
              frame True {
                n294 = local write "Tab Control"(T4."SpotSummary" ("Tab Control")) -> ()
              }
            }
            n295 = local write "Press to goto final Screen"(FALSE ("Press to goto final Screen")) -> ()
            n296 = local write "Output of Spot information"(w404) -> ()
          }
          event "Go Back to Correct": Value Change {
            n297 = event-data() -> ()  [unwired: 1 in, 5 out]
            n298 = local write "Go Back to Correct"(FALSE ("Go Back to Correct")) -> ()
            n299 = local write "Tab Control"(T4."Name and Postions" ("Tab Control")) -> ()
          }
          event "Notes:": Value Change {
            n300 = event-data() -> ("NewVal"=w409:string)  [unwired: 1 in, 4 out]
            n301 = local read "Output of Spot information"() -> (w410:T2)
            n302 = Bundle By Name(cluster=w410, "Notes"=w409) -> (w411:T2)
            n303 = local write "Output of Spot information"(w411) -> ()
          }
        }
      }
    }
  }
  n304 = local write "MetaDataAvailable"(FALSE ("MetaDataAvailable")) -> ()
